vi "test DIO Loop Back.vi"(8 "error in (no error)":errorcluster, 11 "TestCase in":refnum<class "Scan Engine System Tests.lvclass">) -> (0 "error out":errorcluster, 3 "TestCase out":refnum<class "Scan Engine System Tests.lvclass">)   [LabVIEW 2016, in "Scan Engine System Tests.lvclass"]
uses:
  Scan Engine System Tests.lvclass
  C:/Users/rzoeller/Documents/ni-official/niveristand-custom-device-testing-tools/VeriStandTestCase/VeriStandTestCase.lvclass
  <vilib>/addons/_JKI Toolkits/VI Tester/TestCase.llb/TestCase.lvclass
  niveristand-custom-device-testing-tools/VeriStandTestCase/VeriStandTestCase.lvclass
  C:/Program Files (x86)/National Instruments/LabVIEW 2016/vi.lib/addons/_JKI Toolkits/VI Tester/TestCase.llb/TestCase.lvclass
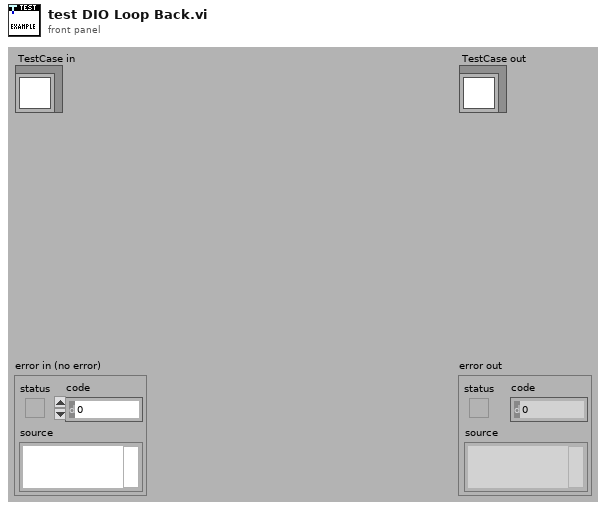
[diagram p1: front panel]
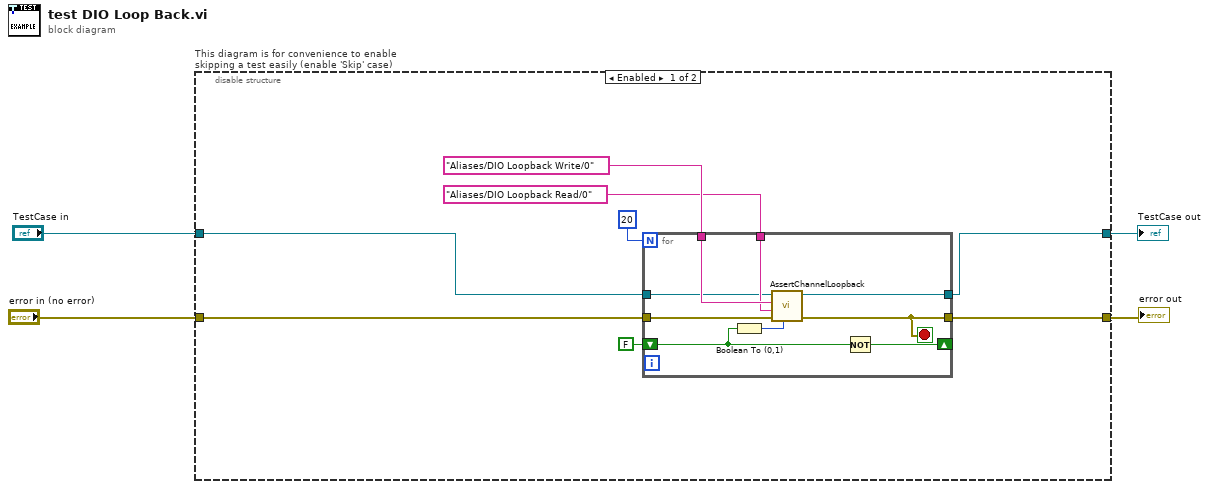
[diagram p0: block diagram]
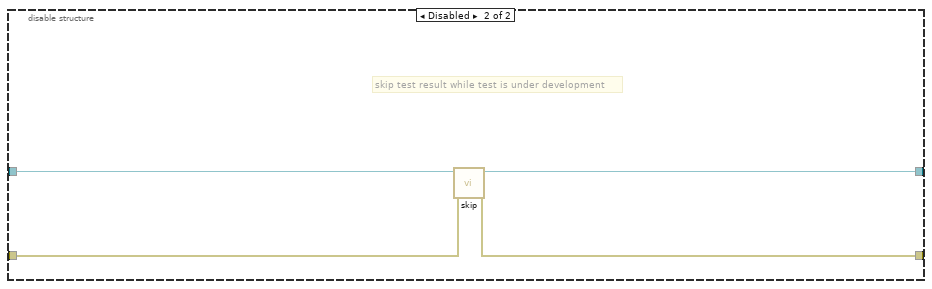
[diagram p2: hidden frame]
diagram:
  n1 = disable-structure "This diagram is for convenience to enable skipping a test easily (enable 'Skip' case)" shown="Enabled" {
    disable-tunnel: "TestCase in" -> [w6 w24]
    disable-tunnel: [w5 w22] -> w1
    disable-tunnel: [w7 w23] -> w3
    disable-tunnel: "error in (no error)" -> [w7 w21]
    frame Enabled {
      n2 = for {
        N: 20 -> [_]
        tunnel: "Aliases/DIO Loopback Write/0" ("Channel") -> [w17]
        tunnel: [w15] -> _
        tunnel: "Aliases/DIO Loopback Read/0" ("Channel") -> [w16]
        shift-right: [w20] -> _
        shift-left: FALSE -> [w19]
        tunnel: w7 -> [w18]
        tunnel: [w12] -> w5
        tunnel: w6 -> [w13]
        stop <- w15 stop-if-true
        n3 = Boolean To (0,1)(Boolean=w19) -> (0, 1=w14:i16)
        n4 = call "AssertChannelLoopback.vi"("Value"=w14, "error in (no error)"=w18, "Read Channel"=w16, "Write Channel"=w17, "VeriStand Test Case in"=w13) -> ("error out"=w15:errorcluster, "VeriStand Test Case out"=w12:refnum<class "Scan Engine System Tests.lvclass">)  [unwired: 5 in]
        n5 = Not(x=w19) -> (.not. x?=w20:bool)
      }
    }
    frame Disabled {
      # "skip test result while test is under development"
      n6 = call <vilib>:"skip.vi"("error in (no error)"=w21, "TestCase in"=w24) -> ("error out"=w23:errorcluster, "TestCase out"=w22:refnum<class "Scan Engine System Tests.lvclass">)  [unwired: 8 in]
    }
  }
  "error out" <- w3
  "TestCase out" <- w1
